vi "Process Image.vi"(8 "error in (no error)":errorcluster, 9 "Quality":i32, 10 "Image Type":T2 items=["Grayscale (U8)", "Grayscale (I16)", "Grayscale (SGL)", "Complex (CSG)", "RGB (U32)", "HSL (U32)", "RGB (U64)", "Grayscale (U16)"], 11 "Image in":T1) -> (0 "error out":errorcluster, 2 "Data String":string, 3 "Image out":T1)   [LabVIEW 2012, in "Image UDP Broadcast Custom Device.lvlib"]
uses:
  Image UDP Broadcast Custom Device.lvlib
  <vilib>/vision/Image Controls.llb/IMAQ Image.ctl
  <vilib>/vision/NI_Vision_Development_Module.lvlib
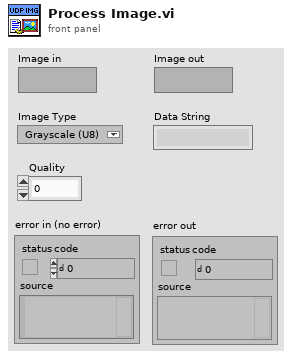
[diagram p1: front panel]
types:
  T1 = typedef "IMAQ Image.ctl" = refnum<image>
  T2 = typedef "Image Type" = u32
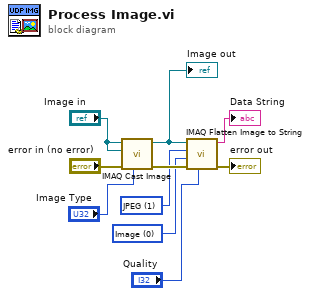
[diagram p0: block diagram]
diagram:
  w4 = 0 items=["Image", "Image and Vision Info", "Reference to Image"] ("Type of Flatten (Image and Vision Info)")
  w3 = 1 items=["None", "JPEG", "PACKED BINARY"] ("Compression (None)")
  n1 = call "IMAQ Cast Image"("Image Type"="Image Type", "error in (no error)"="error in (no error)", "Image Dst"="Image in", "Image Src"="Image in") -> ("error out"=w5:errorcluster, "Image Dst Out"=w8:T1)  [unwired: 6 in]
  "Image out" <- w8
  n2 = call "IMAQ Flatten Image to String"("Quality (750)"="Quality", "error in (no error)"=w5, "Type of Flatten (Image and Vision Info)"=w4, "Compression (None)"=w3, "Image"=w8) -> ("error out"=→"error out":errorcluster, "Data String"=→"Data String":string)  [unwired: 5 in]
